vi "New.vi"(8 "error in (no error)":errorcluster, 9 "Client Key":string, 10 "Secret":string, 11 "Auth ID":string) -> (0 "error out":errorcluster, 3 "WampScramAuthenticator":refnum<class "WampScramAuthenticator.lvclass">)   [LabVIEW 2020, in "wamplv.lvlib" / "WampScramAuthenticator.lvclass"]
uses:
  WampScramAuthenticator.lvclass
  WampScramAuthenticator.lvclass/WampScramAuthenticator.ctl
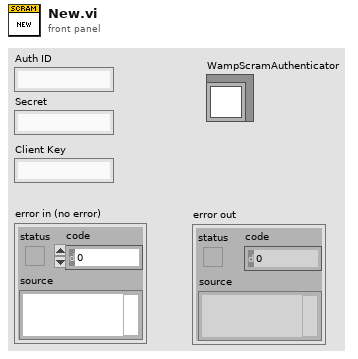
[diagram p1: front panel]
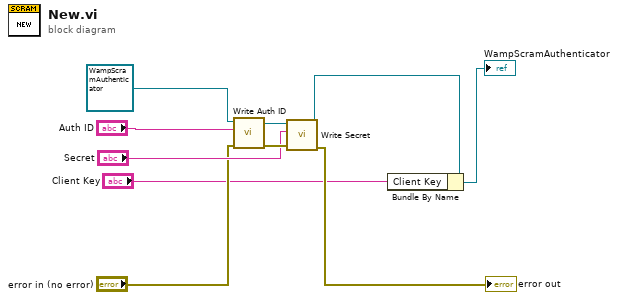
[diagram p0: block diagram]
diagram:
  n1 = call-dynamic "Write Auth ID.vi"("error in (no error)"="error in (no error)", "Auth ID"="Auth ID", "SecretBasedAuthenticatorBase in"=refnum<class "WampScramAuthenticator.lvclass"> refnum ("wamplv.lvlib:WampScramAuthenticator.lvclass")) -> ("error out"=w9:errorcluster, "SecretBasedAuthenticatorBase out"=w10:refnum<class "WampScramAuthenticator.lvclass">)  [unwired: 7 in]
  n2 = call-dynamic "Write Secret.vi"("error in (no error)"=w9, "Secret"="Secret", "SecretBasedAuthenticatorBase in"=w10) -> ("error out"=→"error out":errorcluster, "SecretBasedAuthenticatorBase out"=w3:refnum<class "WampScramAuthenticator.lvclass">)  [unwired: 7 in]
  n3 = Bundle By Name(cluster=w3, "Client Key"="Client Key") -> (→"WampScramAuthenticator":refnum<class "WampScramAuthenticator.lvclass">)
